vi "System6PressureTemp.vi"() -> ()   [LabVIEW 2015]
uses:
  Control 1.ctl
  <vilib>/DAQmx/write.llb/DAQmx Write (Digital 1D Bool NChan 1Samp 1Line).vi
  <vilib>/DAQmx/write.llb/DAQmx Write (Digital Bool 1Line 1Point).vi
  <vilib>/DAQmx/read.llb/DAQmx Read (Analog DBL 1Chan 1Samp).vi
  <vilib>/DAQmx/read.llb/DAQmx Read (Analog 1D Wfm NChan NSamp).vi
  <vilib>/Analysis/baseanly.llb/Mean (DBL).vi
  <vilib>/DAQmx/write.llb/DAQmx Write (Analog DBL 1Chan 1Samp).vi
  <vilib>/DAQmx/miscellaneous.llb/DAQmx Fill In Error Info.vi
  <vilib>/addons/control/pid/NI_PID_autopid.lvlib
  <vilib>/Analysis/NI_AALBase.lvlib
panel:
  out "Voltage Reading(Temp) 2":dbl format="%#_13g"
  out "Temperature (Celcius) 2":dbl format="%#.1g"
  out "Temp(C) 2":dbl(slide) scale=-10.0..100.0
  out "Temp Chart 4":waveform(dbl)(graph)
  out "Temp Chart 3":waveform(dbl)(graph)
  out "Temp 2":dbl
  in  "autotuning parameters 4":T1={"controller type"=1, "relay cycles"=3, "relay amplitude"=1.0, "control specification"=2, "PV noise level"=0.1} {"PV noise level" format="%.2f"; "control specification" items=["normal", "fast", "slow"]; "relay amplitude" format="%.2f"; "controller type" items=["PID", "PI", "P"]}
  in  "PID gains 4":T2={"proportional gain (Kc)"=1.0, "integral time (Ti, min)"=0.01, "derivative time (Td, min)"=0.0} {"derivative time (Td, min)" format="%.3f"; "integral time (Ti, min)" format="%.3f"; "proportional gain (Kc)" format="%.3f"}
  out "PID gains out 4":T2={"proportional gain (Kc)"=1.0, "integral time (Ti, min)"=0.01, "derivative time (Td, min)"=0.0} {"derivative time (Td, min)" format="%.3f"; "integral time (Ti, min)" format="%.3f"; "proportional gain (Kc)" format="%.3f"}
  in  "autotune? (F) 4":bool
  in  "reinitialize? (F) 4":bool
  in  "setpoint in C 2":dbl format="%.2f"
  out "Control Value 4":dbl
  out "ms to wait 2":dbl
  in  "Manual Control 4":bool
  in  "Heater On/Off 2":bool
  out "Voltage Reading(Temp)":dbl format="%#_13g"
  out "Temperature (Celcius)":dbl format="%#.1g"
  out "Temp(C)":dbl(slide) scale=-10.0..100.0
  out "Temp Chart":waveform(dbl)(graph)
  out "Temp Chart 2":waveform(dbl)(graph)
  out "Temp":dbl
  in  "autotuning parameters 3":T1={"controller type"=1, "relay cycles"=3, "relay amplitude"=1.0, "control specification"=2, "PV noise level"=0.1} {"PV noise level" format="%.2f"; "control specification" items=["normal", "fast", "slow"]; "relay amplitude" format="%.2f"; "controller type" items=["PID", "PI", "P"]}
  in  "PID gains 3":T2={"proportional gain (Kc)"=1.0, "integral time (Ti, min)"=0.01, "derivative time (Td, min)"=0.0} {"derivative time (Td, min)" format="%.3f"; "integral time (Ti, min)" format="%.3f"; "proportional gain (Kc)" format="%.3f"}
  out "PID gains out 3":T2={"proportional gain (Kc)"=1.0, "integral time (Ti, min)"=0.01, "derivative time (Td, min)"=0.0} {"derivative time (Td, min)" format="%.3f"; "integral time (Ti, min)" format="%.3f"; "proportional gain (Kc)" format="%.3f"}
  in  "autotune? (F) 3":bool
  in  "reinitialize? (F) 3":bool
  in  "setpoint in C":dbl format="%.2f"
  out "Control Value 3":dbl
  out "ms to wait":dbl
  in  "Manual Control 3":bool
  in  "Heater On/Off":bool
  in  "Open/Close (Green)":bool
  in  "Open/Close (Blue)":bool
  in  "Stop program":bool
  in  "On/Off":bool
  in  "Manual Control 2":bool
  in  "Voltage setting 2":dbl format="%#_13g"
  out "Voltage Reading(pressure) 2":dbl format="%#_13g"
  out "Pressure 2":dbl format="%#.3g"
  out "Pressure Chart 2":dbl(graph)
  in  "autotuning parameters 2":T1={"controller type"=1, "relay cycles"=3, "relay amplitude"=1.0, "control specification"=2, "PV noise level"=0.1} {"PV noise level" format="%.2f"; "control specification" items=["normal", "fast", "slow"]; "relay amplitude" format="%.2f"; "controller type" items=["PID", "PI", "P"]}
  in  "PID gains 2":T2={"proportional gain (Kc)"=1.0, "integral time (Ti, min)"=0.01, "derivative time (Td, min)"=0.0} {"derivative time (Td, min)" format="%.3f"; "integral time (Ti, min)" format="%.3f"; "proportional gain (Kc)" format="%.3f"}
  out "PID gains out 2":T2={"proportional gain (Kc)"=1.0, "integral time (Ti, min)"=0.01, "derivative time (Td, min)"=0.0} {"derivative time (Td, min)" format="%.3f"; "integral time (Ti, min)" format="%.3f"; "proportional gain (Kc)" format="%.3f"}
  in  "autotune? (F) 2":bool
  in  "reinitialize? (F) 2":bool
  in  "setpoint in Bar 2":dbl format="%#.5f"
  out "Control Value 2":dbl
  in  "Voltage setting":dbl format="%#_13g"
  in  "Manual Control":bool
  out "Control Value":dbl
  in  "setpoint in Bar":dbl format="%#.5f"
  in  "reinitialize? (F)":bool
  in  "autotune? (F)":bool
  out "PID gains out":T2={"proportional gain (Kc)"=1.0, "integral time (Ti, min)"=0.01, "derivative time (Td, min)"=0.0} {"derivative time (Td, min)" format="%.3f"; "integral time (Ti, min)" format="%.3f"; "proportional gain (Kc)" format="%.3f"}
  in  "PID gains":T2={"proportional gain (Kc)"=1.0, "integral time (Ti, min)"=0.01, "derivative time (Td, min)"=0.0} {"derivative time (Td, min)" format="%.3f"; "integral time (Ti, min)" format="%.3f"; "proportional gain (Kc)" format="%.3f"}
  in  "autotuning parameters":T1={"controller type"=1, "relay cycles"=3, "relay amplitude"=1.0, "control specification"=2, "PV noise level"=0.1} {"PV noise level" format="%.2f"; "control specification" items=["normal", "fast", "slow"]; "relay amplitude" format="%.2f"; "controller type" items=["PID", "PI", "P"]}
  out "Pressure Chart":dbl(graph)
  out "Pressure":dbl format="%#.3g"
  out "Voltage Reading(pressure)":dbl format="%#_13g"
  # "Pressure Vessel 2"
  # "Pressure Vessel 1"
  # "Readings"
  # "Controls"
  # "Readings"
  # "Controls"
  # "PID Settings"
  # "51.12139\n\n0.044676"
  # "Temperature"
  # "Valves"
  # "Pump 3"
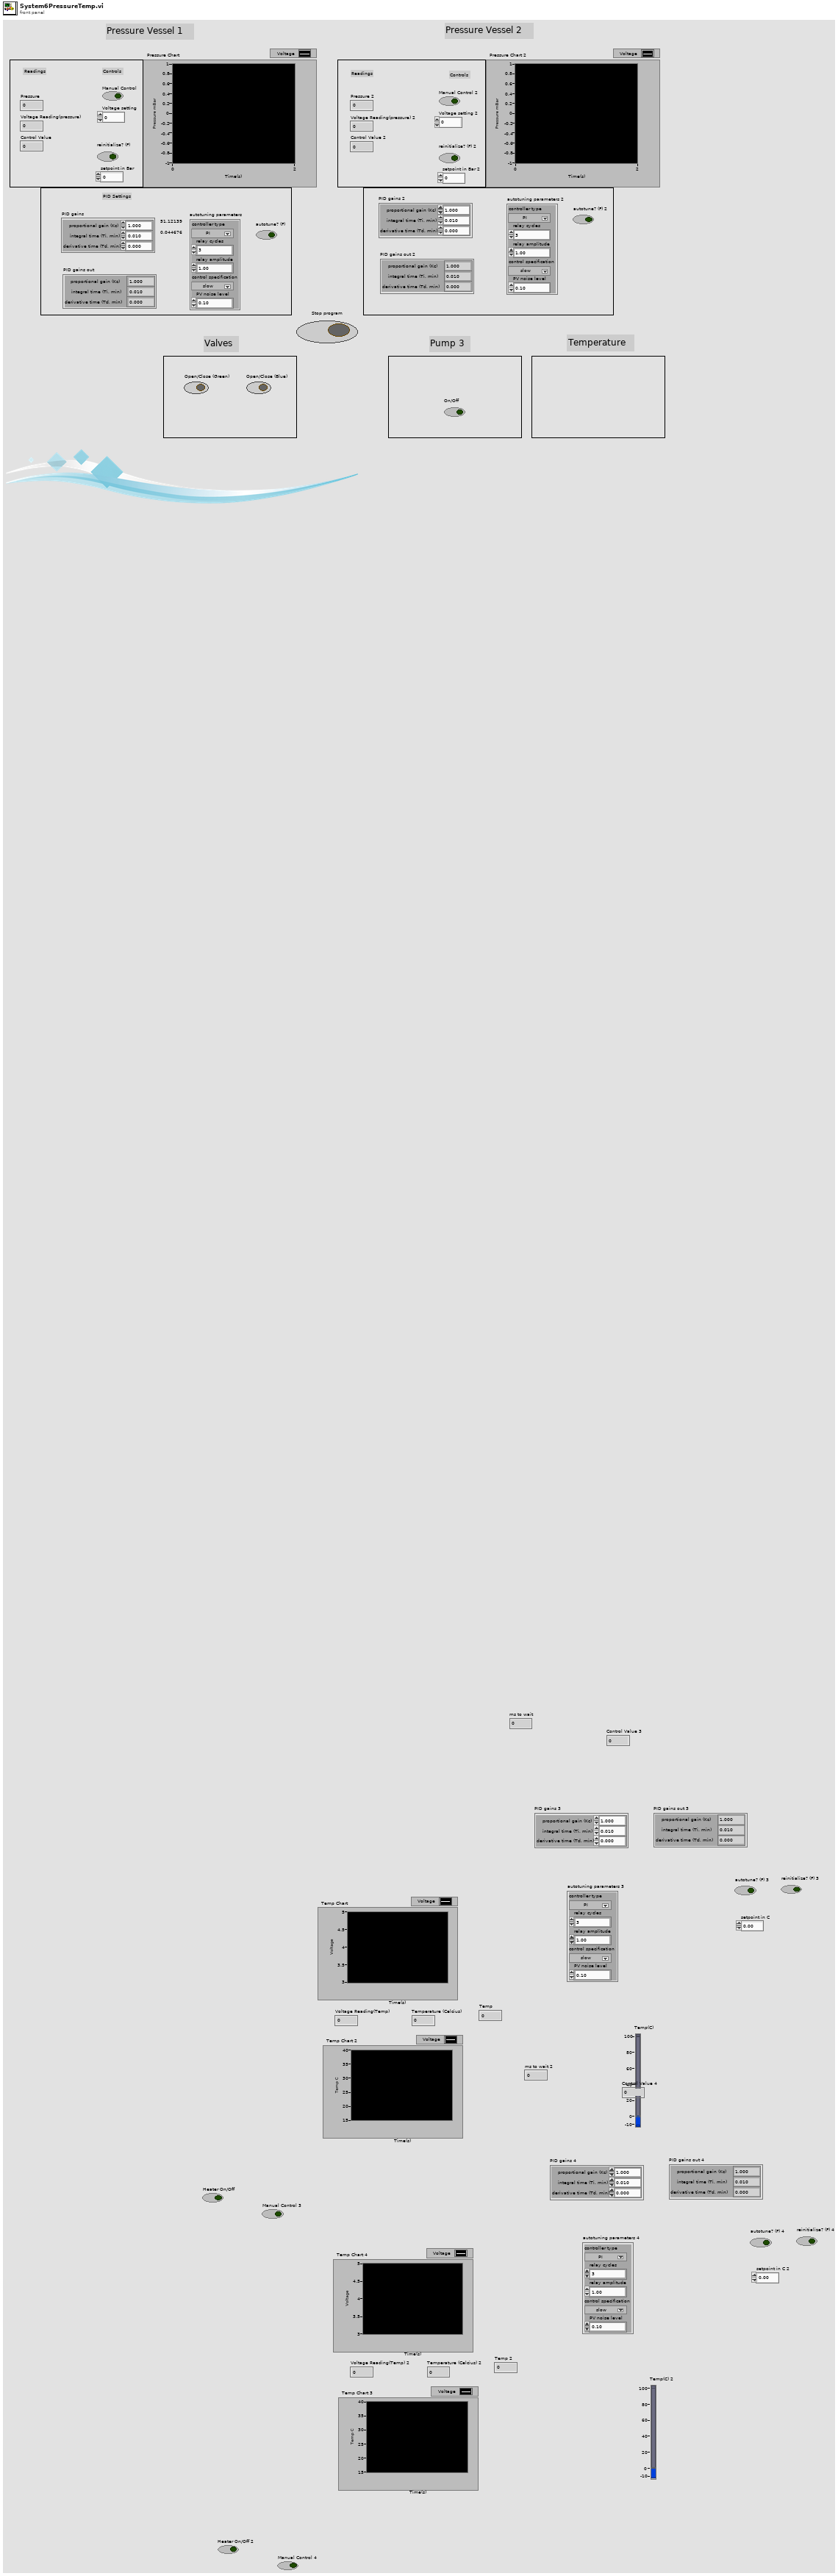
[diagram p1: front panel]
types:
  T1 = cluster{"controller type":u16, "relay cycles":i32, "relay amplitude":dbl, "control specification":u16, "PV noise level":dbl}
  T2 = cluster{"proportional gain (Kc)":dbl, "integral time (Ti, min)":dbl, "derivative time (Td, min)":dbl}
  T3 = typedef "Control 1.ctl" = refnum<k21>
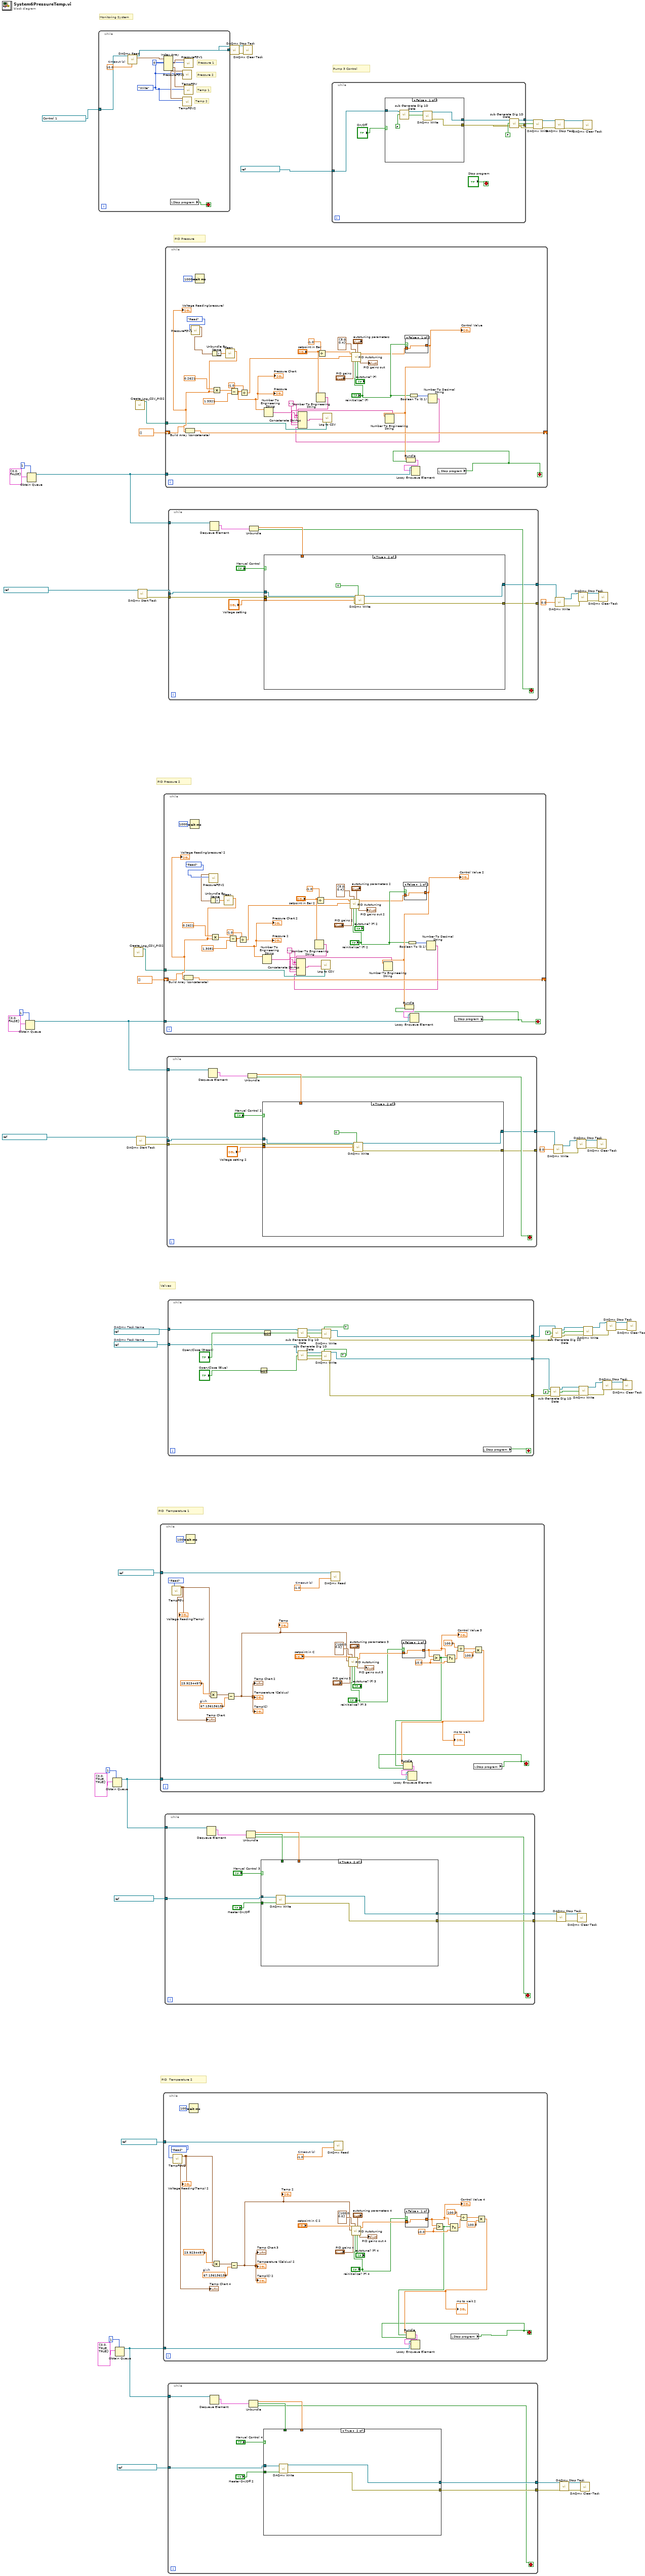
[diagram p0: block diagram]
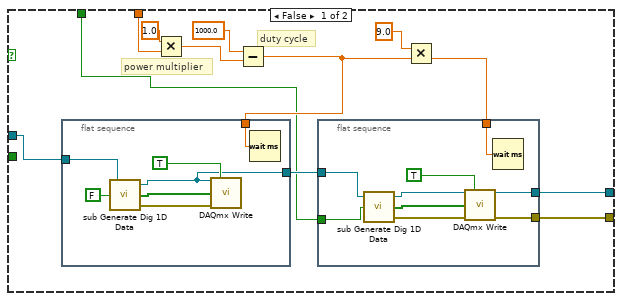
[diagram p2: hidden frame]
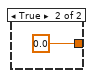
[diagram p3: hidden frame]
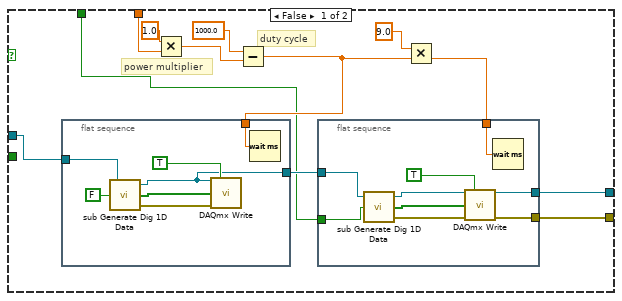
[diagram p4: hidden frame]
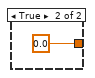
[diagram p5: hidden frame]
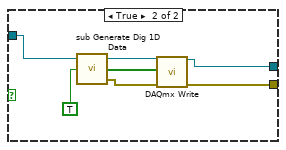
[diagram p6: hidden frame]
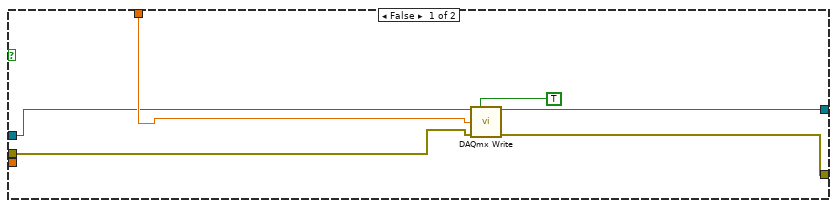
[diagram p7: hidden frame]
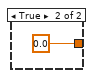
[diagram p8: hidden frame]
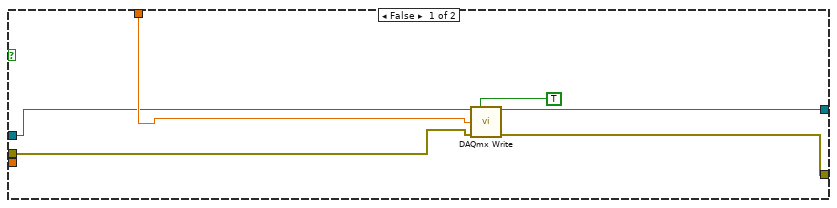
[diagram p9: hidden frame]
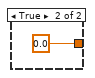
[diagram p10: hidden frame]
diagram:
  w43 = refnum<k21> "NewDigitalSystemBlue"  # DAQmx Task Name
  w44 = refnum<k21> "NewDigitalSystemGreen"  # DAQmx Task Name
  # "Pump 3 Control"
  # "PID  Temperature 2"
  # "PID  Temperature 1"
  # "Monitoring System"
  # "Valves"
  # "PID Pressure"
  # "PID Pressure 2"
  n1 = Obtain Queue(max queue size (-1, unlimited)=1, element data type=cluster{dbl, bool} {0.0, FALSE}) -> (queue out=w68:refnum<queue>)  [unwired: 3 in, 2 out]
  n2 = Obtain Queue(max queue size (-1, unlimited)=1, element data type=cluster{dbl, bool} {0.0, FALSE}) -> (queue out=w82:refnum<queue>)  [unwired: 3 in, 2 out]
  n3 = while {
    tunnel: T3 "New AnalogSystemAI0" -> [w92]
    tunnel: [w91] -> w19
    stop <- w94 stop-if-true
    w84 = enum16{"Write", "Read"}."Write" ("Command")
    w93 = 10.0  # timeout (s)
    # "Temp 2"
    # "Temp 1"
    # "Pressure 2"
    # "Pressure 1"
    n4 = call-poly <vilib>:"DAQmx Read.vi"("task/channels in"=w92, "timeout"=w93) -> ("task out"=w91:refnum<k21>, "data"=w89:waveform(dbl)[])  [unwired: 11 in, 1 out]
    n5 = Index Array(array=w89, index #1=0 ("index")) -> (element #1=w88:waveform(dbl), element #2=w87:waveform(dbl), element #3=w86:waveform(dbl), element #4=w85:waveform(dbl))  [unwired: 3 in]
    n6 = local read "Stop program"() -> (w94:bool)
    n7 = call "PressureFGV2.vi"("Command"=w84, "element"=w87) -> ()  [unwired: 9 in, 1 out]
    n8 = call "TempFGV2.vi"("Command"=w84, "element 3"=w85) -> ()  [unwired: 9 in, 1 out]
    n9 = call "PressureFGV1.vi"("Command"=w84, "element"=w88) -> ()  [unwired: 9 in, 1 out]
    n10 = call "TempFGV.vi"("Command"=w84, "element 3"=w86) -> ()  [unwired: 9 in, 1 out]
  }
  n11 = Obtain Queue(max queue size (-1, unlimited)=1, element data type=cluster{dbl, bool, bool} {0.0, TRUE, TRUE}) -> (queue out=w12:refnum<queue>)  [unwired: 3 in, 2 out]
  n12 = Obtain Queue(max queue size (-1, unlimited)=1, element data type=cluster{dbl, bool, bool} {0.0, TRUE, TRUE}) -> (queue out=w7:refnum<queue>)  [unwired: 3 in, 2 out]
  n13 = call "Create_Log_CSV_PID2.vi"() -> ("path"=w64:path)  [unwired: 11 in]
  n14 = call "Create_Log_CSV_PID2.vi"() -> ("path"=w78:path)  [unwired: 11 in]
  n15 = call <vilib>:"DAQmx Start Task.vi"("task/channels in"=refnum<k21> "NewAnalogSystemAO1") -> ("task out"=w63:refnum<k21>, "error out"=w62:errorcluster)  [unwired: 13 in]
  n16 = call <vilib>:"DAQmx Start Task.vi"("task/channels in"=refnum<k21> "NewAnalogSystemAO0") -> ("task out"=w77:refnum<k21>, "error out"=w76:errorcluster)  [unwired: 13 in]
  n17 = while {
    tunnel: refnum<k21> "MyVoltageTask_0" -> [w118]
    tunnel: w12 -> [w98]
    stop <- w97 stop-if-true
    w104 = 10.0 ("f")
    w119 = 67.136136136  # givh
    w122 = -1.0  # timeout (s)
    n18 = call "TempFGV.vi"("Command"=enum16{"Write", "Read"}."Read") -> ("element 2"=w95:waveform(dbl))  [unwired: 10 in]
    "Voltage Reading(Temp)" <- w95
    "Temp Chart" <- w95
    n19 = Wait (ms)(milliseconds to wait=u32 100) -> ()  [unwired: 1 out]
    n20 = Multiply(x=23.92344976, y=w95) -> (x*y=w120:waveform(dbl))
    n21 = Subtract(x=w120, y=w119) -> (x-y=w102:waveform(dbl))
    "Temperature (Celcius)" <- w102
    "Temp(C)" <- w102
    "Temp Chart 2" <- w102
    "Temp" <- w102
    n22 = call-poly <vilib>:"DAQmx Read.vi"("task/channels in"=w118, "timeout"=w122) -> ()  [unwired: 11 in, 3 out]
    n23 = call <vilib>:"PID Autotuning.vi"("autotune? (F)"="autotune? (F) 3", "autotuning parameters"="autotuning parameters 3", "reinitialize? (F)"="reinitialize? (F) 3", "output range"=cluster{"output high":dbl, "output low":dbl} {"output high"=100.0, "output low"=0.0}, "PID gains"="PID gains 3", "process variable"=w102, "setpoint"="setpoint in C") -> ("PID gains out"=→"PID gains out 3":T2, "output"=w112:dbl)  [unwired: 1 in, 2 out]
    n24 = case shown="False" "reinitialize? (F) 3" {
      tunnel: [w123 0.0] -> w105
      tunnel: w112 -> [w123 _]
      frame False {
      }
      frame True {
      }
    }
    "Control Value 3" <- w105
    n25 = Greater?(x=w105, y=w104) -> (0:w100:bool)
    n26 = Select(t=w105, s=w100, f=w104) -> (s? t:f=w106:dbl)
    n27 = Divide(x=100.0, y=w106) -> (x/y=w108:dbl)
    n28 = local read "Stop program"() -> (w97:bool)
    n29 = Multiply(x=w108, y=100.0) -> (x*y=w101:dbl)
    "ms to wait" <- w101
    n30 = Bundle(w101, w100, "Stop program"=w97) -> (w99:cluster{dbl, bool, "Stop program":bool})  [unwired: 1 in]
    n31 = Lossy Enqueue Element(queue=w98, element=w99) -> ()  [unwired: 1 in, 4 out]
  }
  n32 = while {
    tunnel: refnum<k21> "MyVoltageTask_0" -> [w148]
    tunnel: w7 -> [w128]
    stop <- w125 stop-if-true
    w134 = 10.0 ("f")
    w149 = 67.136136136  # givh
    w152 = -1.0  # timeout (s)
    n33 = call "TempFGV2.vi"("Command"=enum16{"Write", "Read"}."Read") -> ("element 2"=w126:waveform(dbl))  [unwired: 10 in]
    "Voltage Reading(Temp) 2" <- w126
    "Temp Chart 4" <- w126
    n34 = Wait (ms)(milliseconds to wait=u32 100) -> ()  [unwired: 1 out]
    n35 = Multiply(x=23.92344976, y=w126) -> (x*y=w150:waveform(dbl))
    n36 = Subtract(x=w150, y=w149) -> (x-y=w132:waveform(dbl))
    "Temperature (Celcius) 2" <- w132
    "Temp(C) 2" <- w132
    "Temp Chart 3" <- w132
    "Temp 2" <- w132
    n37 = call-poly <vilib>:"DAQmx Read.vi"("task/channels in"=w148, "timeout"=w152) -> ()  [unwired: 11 in, 3 out]
    n38 = call <vilib>:"PID Autotuning.vi"("autotune? (F)"="autotune? (F) 4", "autotuning parameters"="autotuning parameters 4", "reinitialize? (F)"="reinitialize? (F) 4", "output range"=cluster{"output high":dbl, "output low":dbl} {"output high"=100.0, "output low"=0.0}, "PID gains"="PID gains 4", "process variable"=w132, "setpoint"="setpoint in C 2") -> ("PID gains out"=→"PID gains out 4":T2, "output"=w142:dbl)  [unwired: 1 in, 2 out]
    n39 = case shown="False" "reinitialize? (F) 4" {
      tunnel: [w153 0.0] -> w135
      tunnel: w142 -> [w153 _]
      frame False {
      }
      frame True {
      }
    }
    "Control Value 4" <- w135
    n40 = Greater?(x=w135, y=w134) -> (0:w130:bool)
    n41 = Select(t=w135, s=w130, f=w134) -> (s? t:f=w136:dbl)
    n42 = local read "Stop program"() -> (w125:bool)
    n43 = Divide(x=100.0, y=w136) -> (x/y=w138:dbl)
    n44 = Multiply(x=w138, y=100.0) -> (x*y=w131:dbl)
    "ms to wait 2" <- w131
    n45 = Bundle(w131, w130, "Stop program"=w125) -> (w129:cluster{dbl, bool, "Stop program":bool})  [unwired: 1 in]
    n46 = Lossy Enqueue Element(queue=w128, element=w129) -> ()  [unwired: 1 in, 4 out]
  }
  n47 = while {
    tunnel: w68 -> [w181]
    shift-right: [w178] -> _
    shift-left: dbl[] [] -> [w179]
    tunnel: w64 -> [w172]
    stop <- w159 stop-if-true
    w167 = ","
    n48 = Wait (ms)(milliseconds to wait=u32 1000) -> ()  [unwired: 1 out]
    n49 = call "PressureFGV2.vi"("Command"=enum16{"Write", "Read"}."Read") -> ("element 2"=w155:waveform(dbl))  [unwired: 10 in]
    n50 = Unbundle By Name(w155) -> ("Y"=w157:dbl[])
    n51 = call-poly <vilib>:"Mean.vi"("X"=w157) -> ("mean"=w180:dbl)  [unwired: 1 out]
    "Voltage Reading(pressure) 2" <- w180
    n52 = Build Array (concatenate)(w179, w180) -> (w178:dbl[])
    n53 = Multiply(x=0.2621, y=w180) -> (x*y=w188:dbl)
    n54 = Subtract(x=w188, y=1.3081) -> (x-y=w176:dbl)
    "Pressure 2" <- w176
    "Pressure Chart 2" <- w176
    n55 = Divide(x=w176, y=-1.0) -> (x/y=w164:dbl)
    n56 = Number To Engineering String(4:w176) -> (0:w171:string)  [unwired: 3 in]
    n57 = Number To Engineering String(4:"setpoint in Bar 2") -> (0:w170:string)  [unwired: 3 in]
    n58 = Divide(x="setpoint in Bar 2", y=-1.0) -> (x/y=w163:dbl)
    n59 = call <vilib>:"PID Autotuning.vi"("autotune? (F)"="autotune? (F) 2", "autotuning parameters"="autotuning parameters 2", "reinitialize? (F)"="reinitialize? (F) 2", "output range"=cluster{"output high":dbl, "output low":dbl} {"output high"=5.0, "output low"=0.4}, "PID gains"="PID gains 2", "process variable"=w164, "setpoint"=w163) -> ("PID gains out"=→"PID gains out 2":T2, "output"=w161:dbl)  [unwired: 1 in, 2 out]
    n60 = case shown="False" "reinitialize? (F) 2" {
      tunnel: [w190 0.0] -> w175
      tunnel: w161 -> [w190 _]
      frame False {
      }
      frame True {
      }
    }
    "Control Value 2" <- w175
    n61 = Number To Engineering String(4:w175) -> (0:w174:string)  [unwired: 3 in]
    n62 = Boolean To (0,1)(Boolean="reinitialize? (F) 2") -> (0, 1=w168:i16)
    n63 = Number To Decimal String(number=w168) -> (decimal integer string=w166:string)  [unwired: 1 in]
    n64 = Concatenate Strings(w170, w167, w171, w167, w174, w167, w166) -> (w173:string)
    n65 = call "Log to CSV.vi"("Data Str"=w173, "Path"=w172) -> ()  [unwired: 5 in, 1 out]
    n66 = local read "Stop program"() -> (w159:bool)
    n67 = Bundle("output"=w175, "Stop program"=w159) -> (w160:cluster{"output":dbl, "Stop program":bool})  [unwired: 1 in]
    n68 = Lossy Enqueue Element(queue=w181, element=w160) -> ()  [unwired: 1 in, 4 out]
  }
  n69 = while {
    tunnel: w12 -> [w201]
    tunnel: refnum<k21> "MyDigitalOutTask_2" -> [w198]
    tunnel: [w194] -> w15
    tunnel: [w193] -> w16
    stop <- w192 stop-if-true
    n70 = Dequeue Element(queue=w201) -> (element=w197:cluster{dbl, bool, bool})  [unwired: 2 in, 3 out]
    n71 = Unbundle(w197) -> (w196:dbl, w195:bool, w192:bool)
    n72 = case shown="True" "Manual Control 3" {
      tunnel: w198 -> [w212 w233]
      tunnel: "Heater On/Off" -> [_ w232]
      tunnel: w196 -> [w211 _]
      tunnel: w195 -> [w206 _]
      tunnel: [w203 w231] -> w194
      tunnel: [w202 w230] -> w193
      frame False {
        # "duty cycle"
        # "power multiplier"
        n73 = flat-sequence {
          tunnel: w212 -> [w226]
          tunnel: [w225] -> w213
          tunnel: w210 -> [w224]
          frame #0 {
            n74 = call <vilib>:"sub Generate Dig 1D Data.vi"("initial value"=FALSE, "task in"=w226) -> ("error out"=w228:errorcluster, "Data"=w229:bool[], "task out"=w225:refnum<k21>)  [unwired: 1 in]
            n75 = call-poly <vilib>:"DAQmx Write.vi"("task/channels in"=w225, "auto start"=TRUE, "data"=w229, "error in"=w228) -> ()  [unwired: 9 in, 3 out]
            n76 = Wait (ms)(milliseconds to wait=w224) -> ()  [unwired: 1 out]
          }
        }
        n77 = Multiply(x=1.0, y=w211) -> (x*y=w205:dbl)
        n78 = Subtract(x=1000.0, y=w205) -> (x-y=w210:dbl)
        n79 = flat-sequence {
          tunnel: w213 -> [w218]
          tunnel: w208 -> [w217]
          tunnel: w206 -> [w216]
          tunnel: [w215] -> w203
          tunnel: [w214] -> w202
          frame #0 {
            n80 = call <vilib>:"sub Generate Dig 1D Data.vi"("initial value"=w216, "task in"=w218) -> ("error out"=w221:errorcluster, "Data"=w219:bool[], "task out"=w220:refnum<k21>)  [unwired: 1 in]
            n81 = call-poly <vilib>:"DAQmx Write.vi"("task/channels in"=w220, "auto start"=TRUE, "data"=w219, "error in"=w221) -> ("task out"=w215:refnum<k21>, "error out"=w214:errorcluster)  [unwired: 9 in, 1 out]
            n82 = Wait (ms)(milliseconds to wait=w217) -> ()  [unwired: 1 out]
          }
        }
        n83 = Multiply(x=9.0, y=w210) -> (x*y=w208:dbl)
      }
      frame True {
        n84 = call-poly <vilib>:"DAQmx Write.vi"("task/channels in"=w233, "data"=w232) -> ("task out"=w231:refnum<k21>, "error out"=w230:errorcluster)  [unwired: 11 in, 1 out]
      }
    }
  }
  n85 = while {
    tunnel: w82 -> [w260]
    shift-right: [w255] -> _
    shift-left: dbl[] [] -> [w256]
    tunnel: w78 -> [w249]
    stop <- w237 stop-if-true
    w244 = ","
    n86 = call "PressureFGV1.vi"("Command"=enum16{"Write", "Read"}."Read") -> ("element 2"=w234:waveform(dbl))  [unwired: 10 in]
    n87 = Wait (ms)(milliseconds to wait=u32 1000) -> ()  [unwired: 1 out]
    n88 = Unbundle By Name(w234) -> ("Y"=w258:dbl[])
    n89 = call-poly <vilib>:"Mean.vi"("X"=w258) -> ("mean"=w257:dbl)  [unwired: 1 out]
    "Voltage Reading(pressure)" <- w257
    n90 = Build Array (concatenate)(w256, w257) -> (w255:dbl[])
    n91 = Multiply(x=0.2621, y=w257) -> (x*y=w267:dbl)
    n92 = Subtract(x=w267, y=1.3321) -> (x-y=w253:dbl)
    "Pressure" <- w253
    "Pressure Chart" <- w253
    n93 = Divide(x=w253, y=-1.0) -> (x/y=w241:dbl)
    n94 = Number To Engineering String(4:w253) -> (0:w248:string)  [unwired: 3 in]
    n95 = Number To Engineering String(4:"setpoint in Bar") -> (0:w247:string)  [unwired: 3 in]
    n96 = Divide(x="setpoint in Bar", y=-1.0) -> (x/y=w240:dbl)
    n97 = call <vilib>:"PID Autotuning.vi"("autotune? (F)"="autotune? (F)", "autotuning parameters"="autotuning parameters", "reinitialize? (F)"="reinitialize? (F)", "output range"=cluster{"output high":dbl, "output low":dbl} {"output high"=5.0, "output low"=0.4}, "PID gains"="PID gains", "process variable"=w241, "setpoint"=w240) -> ("PID gains out"=→"PID gains out":T2, "output"=w238:dbl)  [unwired: 1 in, 2 out]
    n98 = case shown="False" "reinitialize? (F)" {
      tunnel: [w269 0.0] -> w252
      tunnel: w238 -> [w269 _]
      frame False {
      }
      frame True {
      }
    }
    "Control Value" <- w252
    n99 = Number To Engineering String(4:w252) -> (0:w251:string)  [unwired: 3 in]
    n100 = Boolean To (0,1)(Boolean="reinitialize? (F)") -> (0, 1=w245:i16)
    n101 = Number To Decimal String(number=w245) -> (decimal integer string=w243:string)  [unwired: 1 in]
    n102 = Concatenate Strings(w247, w244, w248, w244, w251, w244, w243) -> (w250:string)
    n103 = call "Log to CSV.vi"("Data Str"=w250, "Path"=w249) -> ()  [unwired: 5 in, 1 out]
    n104 = local read "Stop program"() -> (w237:bool)
    n105 = Bundle("output"=w252, "Stop program"=w237) -> (w259:cluster{"output":dbl, "Stop program":bool})  [unwired: 1 in]
    n106 = Lossy Enqueue Element(queue=w260, element=w259) -> ()  [unwired: 1 in, 4 out]
  }
  n107 = while {
    tunnel: w68 -> [w280]
    tunnel: w63 -> [w278]
    tunnel: [w273] -> w60
    tunnel: w62 -> [w272]
    tunnel: [w271] -> _
    stop <- w274 stop-if-true
    n108 = Dequeue Element(queue=w280) -> (element=w277:cluster{dbl, bool})  [unwired: 2 in, 3 out]
    n109 = Unbundle(w277) -> (w276:dbl, w274:bool)
    n110 = case shown="True" "Manual Control 2" {
      tunnel: w278 -> [w284 w291]
      tunnel: w276 -> [w285 _]
      tunnel: "Voltage setting 2" -> [_ w290]
      tunnel: [w283 w289] -> w273
      tunnel: w272 -> [w282 w288]
      tunnel: [w281 w287] -> w271
      frame False {
        n111 = call-poly <vilib>:"DAQmx Write.vi"("task/channels in"=w284, "auto start"=TRUE, "data"=w285, "error in"=w282) -> ("task out"=w283:refnum<k21>, "error out"=w281:errorcluster)  [unwired: 9 in, 1 out]
      }
      frame True {
        n112 = call-poly <vilib>:"DAQmx Write.vi"("task/channels in"=w291, "auto start"=TRUE, "data"=w290, "error in"=w288) -> ("task out"=w289:refnum<k21>, "error out"=w287:errorcluster)  [unwired: 9 in, 1 out]
      }
    }
  }
  n113 = while {
    tunnel: w44 -> [w301]
    tunnel: w43 -> [w300]
    tunnel: [w299] -> w33
    tunnel: [w298] -> w29
    tunnel: [w295] -> w26
    tunnel: [w294] -> w24
    stop <- w293 stop-if-true
    n114 = Not(x="Open/Close (Blue)") -> (.not. x?=w311:bool)
    n115 = Not(x="Open/Close (Green)") -> (.not. x?=w310:bool)
    n116 = call <vilib>:"sub Generate Dig 1D Data.vi"("initial value"=w310, "task in"=w301) -> ("error out"=w297:errorcluster, "Data"=w308:bool[], "task out"=w305:refnum<k21>)  [unwired: 1 in]
    n117 = call <vilib>:"sub Generate Dig 1D Data.vi"("initial value"=w311, "task in"=w300) -> ("error out"=w296:errorcluster, "Data"=w307:bool[], "task out"=w306:refnum<k21>)  [unwired: 1 in]
    n118 = call-poly <vilib>:"DAQmx Write.vi"("task/channels in"=w305, "auto start"=TRUE, "data"=w308, "error in"=w297) -> ("task out"=w299:refnum<k21>, "error out"=w295:errorcluster)  [unwired: 9 in, 1 out]
    n119 = call-poly <vilib>:"DAQmx Write.vi"("task/channels in"=w306, "auto start"=TRUE, "data"=w307, "error in"=w296) -> ("task out"=w298:refnum<k21>, "error out"=w294:errorcluster)  [unwired: 9 in, 1 out]
    n120 = local read "Stop program"() -> (w293:bool)
  }
  n121 = while {
    tunnel: w7 -> [w321]
    tunnel: refnum<k21> "MyDigitalOutTask_2" -> [w318]
    tunnel: [w314] -> w4
    tunnel: [w313] -> w3
    stop <- w312 stop-if-true
    n122 = Dequeue Element(queue=w321) -> (element=w317:cluster{dbl, bool, bool})  [unwired: 2 in, 3 out]
    n123 = Unbundle(w317) -> (w316:dbl, w315:bool, w312:bool)
    n124 = case shown="True" "Manual Control 4" {
      tunnel: w318 -> [w332 w353]
      tunnel: "Heater On/Off 2" -> [_ w352]
      tunnel: w316 -> [w331 _]
      tunnel: w315 -> [w326 _]
      tunnel: [w323 w351] -> w314
      tunnel: [w322 w350] -> w313
      frame False {
        # "duty cycle"
        # "power multiplier"
        n125 = flat-sequence {
          tunnel: w332 -> [w346]
          tunnel: [w345] -> w333
          tunnel: w330 -> [w344]
          frame #0 {
            n126 = call <vilib>:"sub Generate Dig 1D Data.vi"("initial value"=FALSE, "task in"=w346) -> ("error out"=w348:errorcluster, "Data"=w349:bool[], "task out"=w345:refnum<k21>)  [unwired: 1 in]
            n127 = call-poly <vilib>:"DAQmx Write.vi"("task/channels in"=w345, "auto start"=TRUE, "data"=w349, "error in"=w348) -> ()  [unwired: 9 in, 3 out]
            n128 = Wait (ms)(milliseconds to wait=w344) -> ()  [unwired: 1 out]
          }
        }
        n129 = Multiply(x=1.0, y=w331) -> (x*y=w325:dbl)
        n130 = Subtract(x=1000.0, y=w325) -> (x-y=w330:dbl)
        n131 = flat-sequence {
          tunnel: w333 -> [w338]
          tunnel: w328 -> [w337]
          tunnel: w326 -> [w336]
          tunnel: [w335] -> w323
          tunnel: [w334] -> w322
          frame #0 {
            n132 = call <vilib>:"sub Generate Dig 1D Data.vi"("initial value"=w336, "task in"=w338) -> ("error out"=w341:errorcluster, "Data"=w339:bool[], "task out"=w340:refnum<k21>)  [unwired: 1 in]
            n133 = call-poly <vilib>:"DAQmx Write.vi"("task/channels in"=w340, "auto start"=TRUE, "data"=w339, "error in"=w341) -> ("task out"=w335:refnum<k21>, "error out"=w334:errorcluster)  [unwired: 9 in, 1 out]
            n134 = Wait (ms)(milliseconds to wait=w337) -> ()  [unwired: 1 out]
          }
        }
        n135 = Multiply(x=9.0, y=w330) -> (x*y=w328:dbl)
      }
      frame True {
        n136 = call-poly <vilib>:"DAQmx Write.vi"("task/channels in"=w353, "data"=w352) -> ("task out"=w351:refnum<k21>, "error out"=w350:errorcluster)  [unwired: 11 in, 1 out]
      }
    }
  }
  n137 = while {
    tunnel: w82 -> [w363]
    tunnel: w77 -> [w361]
    tunnel: [w356] -> w74
    tunnel: w76 -> [w355]
    tunnel: [w354] -> _
    stop <- w357 stop-if-true
    n138 = Dequeue Element(queue=w363) -> (element=w360:cluster{dbl, bool})  [unwired: 2 in, 3 out]
    n139 = Unbundle(w360) -> (w359:dbl, w357:bool)
    n140 = case shown="True" "Manual Control" {
      tunnel: w361 -> [w367 w374]
      tunnel: w359 -> [w368 _]
      tunnel: "Voltage setting" -> [_ w373]
      tunnel: [w366 w372] -> w356
      tunnel: w355 -> [w365 w371]
      tunnel: [w364 w370] -> w354
      frame False {
        n141 = call-poly <vilib>:"DAQmx Write.vi"("task/channels in"=w367, "auto start"=TRUE, "data"=w368, "error in"=w365) -> ("task out"=w366:refnum<k21>, "error out"=w364:errorcluster)  [unwired: 9 in, 1 out]
      }
      frame True {
        n142 = call-poly <vilib>:"DAQmx Write.vi"("task/channels in"=w374, "auto start"=TRUE, "data"=w373, "error in"=w371) -> ("task out"=w372:refnum<k21>, "error out"=w370:errorcluster)  [unwired: 9 in, 1 out]
      }
    }
  }
  n143 = call <vilib>:"DAQmx Stop Task.vi"("task/channels in"=w19) -> ("task out"=w21:refnum<k21>, "error out"=w20:errorcluster)  [unwired: 13 in]
  n144 = call <vilib>:"DAQmx Clear Task.vi"("task in"=w21, "error in"=w20) -> ()  [unwired: 13 in, 1 out]
  n145 = while {
    tunnel: refnum<k21> "NewDigSystemP0L2" -> [w379]
    tunnel: [w378] -> w48
    tunnel: [w377] -> w47
    stop <- "Stop program" stop-if-true
    n146 = case shown="False" "On/Off" {
      tunnel: w379 -> [w386 w390]
      tunnel: [w382 w389] -> w378
      tunnel: [w381 w387] -> w377
      frame False {
        n147 = call <vilib>:"sub Generate Dig 1D Data.vi"("initial value"=FALSE, "task in"=w386) -> ("Data"=w384:bool[], "task out"=w385:refnum<k21>)  [unwired: 1 in, 1 out]
        n148 = call-poly <vilib>:"DAQmx Write.vi"("task/channels in"=w385, "data"=w384) -> ("task out"=w382:refnum<k21>, "error out"=w381:errorcluster)  [unwired: 11 in, 1 out]
      }
      frame True {
        n149 = call <vilib>:"sub Generate Dig 1D Data.vi"("initial value"=TRUE, "task in"=w390) -> ("error out"=w388:errorcluster, "Data"=w392:bool[], "task out"=w391:refnum<k21>)  [unwired: 1 in]
        n150 = call-poly <vilib>:"DAQmx Write.vi"("task/channels in"=w391, "data"=w392, "error in"=w388) -> ("task out"=w389:refnum<k21>, "error out"=w387:errorcluster)  [unwired: 10 in, 1 out]
      }
    }
  }
  n151 = call <vilib>:"sub Generate Dig 1D Data.vi"("error in"=w47, "initial value"=FALSE, "task in"=w48) -> ("error out"=w52:errorcluster, "Data"=w50:bool[], "task out"=w51:refnum<k21>)
  n152 = call-poly <vilib>:"DAQmx Write.vi"("task/channels in"=w51, "data"=w50, "error in"=w52) -> ("task out"=w46:refnum<k21>, "error out"=w45:errorcluster)  [unwired: 10 in, 1 out]
  n153 = call <vilib>:"sub Generate Dig 1D Data.vi"("error in"=w24, "initial value"=FALSE, "task in"=w29) -> ("error out"=w23:errorcluster, "Data"=w28:bool[], "task out"=w30:refnum<k21>)
  n154 = call <vilib>:"sub Generate Dig 1D Data.vi"("error in"=w26, "initial value"=FALSE, "task in"=w33) -> ("error out"=w25:errorcluster, "Data"=w27:bool[], "task out"=w34:refnum<k21>)
  n155 = call-poly <vilib>:"DAQmx Write.vi"("task/channels in"=w60, "data"=0.0) -> ("task out"=w59:refnum<k21>, "error out"=w58:errorcluster)  [unwired: 11 in, 1 out]
  n156 = call-poly <vilib>:"DAQmx Write.vi"("task/channels in"=w74, "data"=0.0) -> ("task out"=w73:refnum<k21>, "error out"=w72:errorcluster)  [unwired: 11 in, 1 out]
  n157 = call <vilib>:"DAQmx Stop Task.vi"("task/channels in"=w46, "error in"=w45) -> ("task out"=w54:refnum<k21>, "error out"=w53:errorcluster)  [unwired: 12 in]
  n158 = call <vilib>:"DAQmx Stop Task.vi"("task/channels in"=w15, "error in"=w16) -> ("task out"=w17:refnum<k21>, "error out"=w18:errorcluster)  [unwired: 12 in]
  n159 = call <vilib>:"DAQmx Stop Task.vi"("task/channels in"=w4, "error in"=w3) -> ("task out"=w2:refnum<k21>, "error out"=w1:errorcluster)  [unwired: 12 in]
  n160 = call <vilib>:"DAQmx Stop Task.vi"("task/channels in"=w59, "error in"=w58) -> ("task out"=w61:refnum<k21>, "error out"=w57:errorcluster)  [unwired: 12 in]
  n161 = call <vilib>:"DAQmx Clear Task.vi"("task in"=w17, "error in"=w18) -> ()  [unwired: 13 in, 1 out]
  n162 = call <vilib>:"DAQmx Stop Task.vi"("task/channels in"=w73, "error in"=w72) -> ("task out"=w75:refnum<k21>, "error out"=w71:errorcluster)  [unwired: 12 in]
  n163 = call-poly <vilib>:"DAQmx Write.vi"("task/channels in"=w30, "data"=w28, "error in"=w23) -> ("task out"=w37:refnum<k21>, "error out"=w36:errorcluster)  [unwired: 10 in, 1 out]
  n164 = call <vilib>:"DAQmx Clear Task.vi"("task in"=w2, "error in"=w1) -> ()  [unwired: 13 in, 1 out]
  n165 = call <vilib>:"DAQmx Clear Task.vi"("task in"=w54, "error in"=w53) -> ()  [unwired: 13 in, 1 out]
  n166 = call-poly <vilib>:"DAQmx Write.vi"("task/channels in"=w34, "data"=w27, "error in"=w25) -> ("task out"=w40:refnum<k21>, "error out"=w41:errorcluster)  [unwired: 10 in, 1 out]
  n167 = call <vilib>:"DAQmx Clear Task.vi"("task in"=w61, "error in"=w57) -> ()  [unwired: 13 in, 1 out]
  n168 = call <vilib>:"DAQmx Clear Task.vi"("task in"=w75, "error in"=w71) -> ()  [unwired: 13 in, 1 out]
  n169 = call <vilib>:"DAQmx Stop Task.vi"("task/channels in"=w37, "error in"=w36) -> ("task out"=w38:refnum<k21>, "error out"=w35:errorcluster)  [unwired: 12 in]
  n170 = call <vilib>:"DAQmx Stop Task.vi"("task/channels in"=w40, "error in"=w41) -> ("task out"=w39:refnum<k21>, "error out"=w42:errorcluster)  [unwired: 12 in]
  n171 = call <vilib>:"DAQmx Clear Task.vi"("task in"=w38, "error in"=w35) -> ()  [unwired: 13 in, 1 out]
  n172 = call <vilib>:"DAQmx Clear Task.vi"("task in"=w39, "error in"=w42) -> ()  [unwired: 13 in, 1 out]
